vi "Init.vi"(8 "error in (no error)":errorcluster, 11 "Submission Data":T1) -> (0 "error out":errorcluster, 3 "Submission out":refnum<class "Submission.lvclass">)   [LabVIEW 2020, in "Summer of LabVIEW.lvlib" / "Submission.lvclass"]
uses:
  Submission.lvclass
  Submission.lvclass/Submission.ctl
  SoL Scoring/Score Entry.ctl
  SoL Scoring/SoL Scoring.lvlib
  SoL Scoring/Score.ctl
  Submission Data.ctl
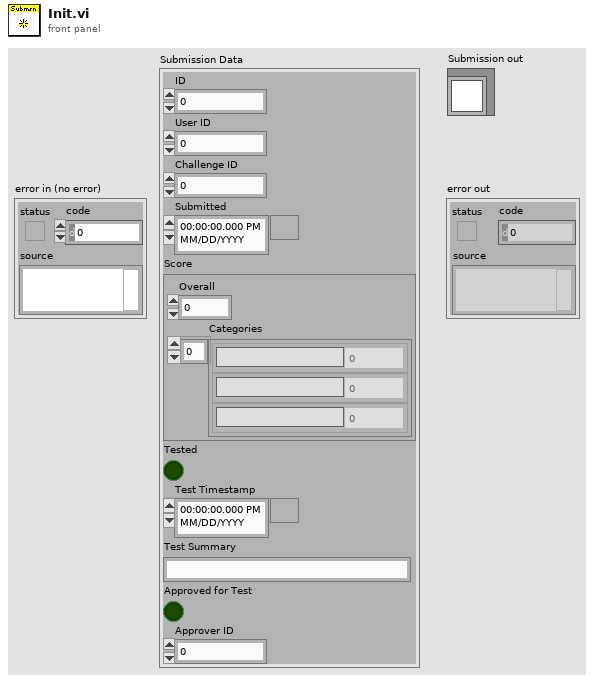
[diagram p1: front panel]
types:
  T1 = typedef "Summer of LabVIEW.lvlib/Submission.lvclass/Submission Data.ctl" = cluster{"ID":i64, "User ID":i64, "Challenge ID":i64, "Submitted":timestamp, "Score":T2, "Tested":bool, "Test Timestamp":timestamp, "Test Summary":string, "Approved for Test":bool, "Approver ID":i64}
  T2 = typedef "SoL Scoring.lvlib/Score.ctl" = cluster{"Overall":dbl, "Categories":T3[]}
  T3 = typedef "SoL Scoring.lvlib/Score Entry.ctl" = cluster{"Category":string, "Value":dbl}
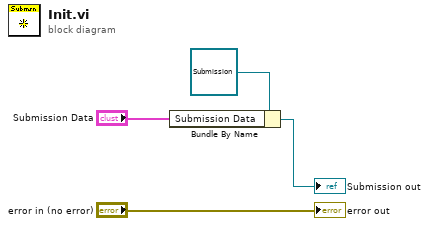
[diagram p0: block diagram]
diagram:
  n1 = Bundle By Name(cluster=refnum<class "Submission.lvclass"> refnum ("Submission in"), "Submission Data"="Submission Data") -> (→"Submission out":refnum<class "Submission.lvclass">)
  "error out" <- "error in (no error)"
